vi "Init Plot Toolbar.vi"(8 "error in (no error)":errorcluster, 11 "Refs":T1) -> (0 "error out":errorcluster, 3 "Refs (dup)":T1)   [LabVIEW 2021, in "RocketPlot.lvlib"]
uses:
  RocketPlot.lvlib
  TypeDefs/Plot UI references.ctl
  Classes/RocketPlotHandle/RocketPlotHandle.lvclass
  <userlib>/bjustice/TipStripOOPanel/Classes/TipPanelHandle/TipPanelHandle.lvclass
  TypeDefs/Plot top row.ctl
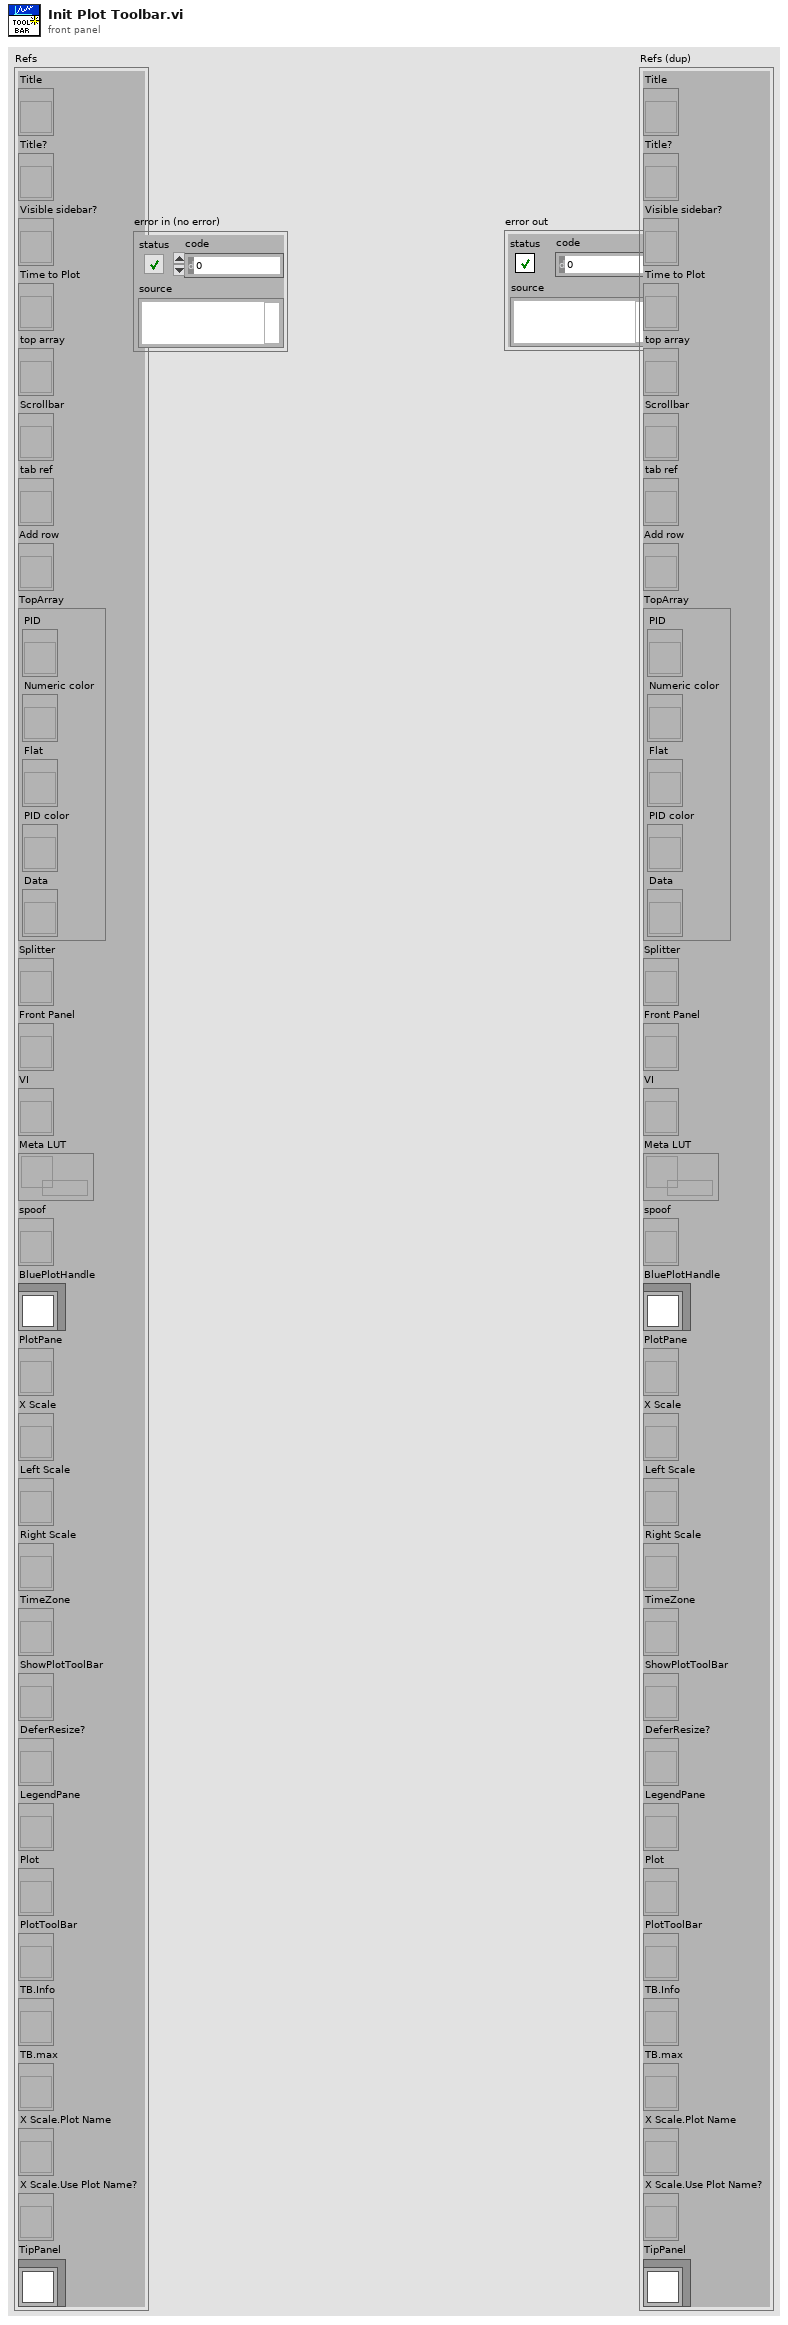
[diagram p1: front panel]
types:
  T1 = typedef "RocketPlot.lvlib/Plot UI references.ctl" = cluster{"Title":refnum<vi>, "Title?":refnum<vi>, "Visible sidebar?":refnum<vi>, "Time to Plot":refnum<vi>, "top array":refnum<vi>, "Scrollbar":refnum<vi>, "tab ref":refnum<vi>, "Add row":refnum<vi>, "TopArray":cluster{"PID":refnum<vi>, "Numeric color":refnum<vi>, "Flat":refnum<vi>, "PID color":refnum<vi>, "Data":refnum<vi>}, "Splitter":refnum<vi>, "Front Panel":refnum<vi>, "VI":refnum<vi>, "Meta LUT":refnum<data-value>, "spoof":refnum<vi>, "BluePlotHandle":refnum<class "RocketPlotHandle.lvclass">, "PlotPane":refnum<vi>, "X Scale":refnum<vi>, "Left Scale":refnum<vi>, "Right Scale":refnum<vi>, "TimeZone":refnum<vi>, "ShowPlotToolBar":refnum<vi>, "DeferResize?":refnum<vi>, "LegendPane":refnum<vi>, "Plot":refnum<vi>, "PlotToolBar":refnum<vi>, "TB.Info":refnum<vi>, "TB.max":refnum<vi>, "X Scale.Plot Name":refnum<vi>, "X Scale.Use Plot Name?":refnum<vi>, "TipPanel":refnum<class "TipPanelHandle.lvclass">}
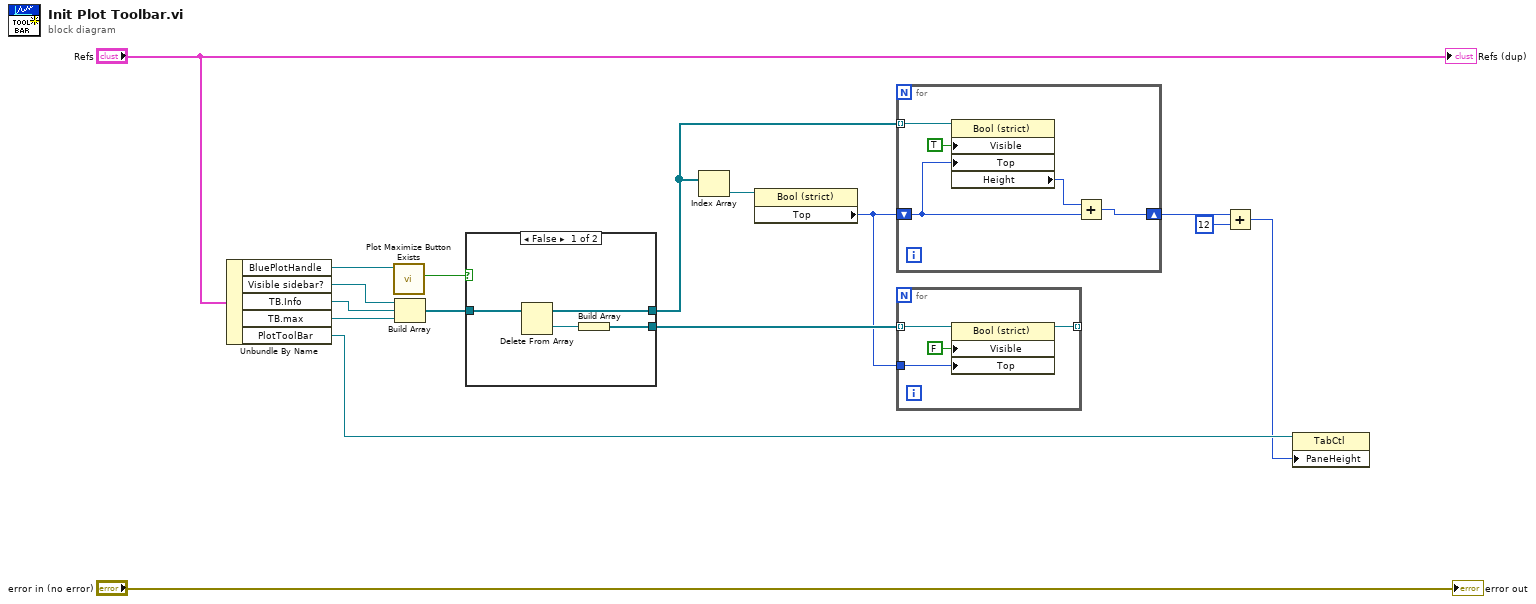
[diagram p0: block diagram]
diagram:
  n1 = Unbundle By Name("Refs") -> ("BluePlotHandle"=w12:refnum<class "RocketPlotHandle.lvclass">, "Visible sidebar?"=w15:refnum<vi>, "TB.Info"=w14:refnum<vi>, "TB.max"=w13:refnum<vi>, "PlotToolBar"=w4:refnum<vi>)
  n2 = call-dynamic "Plot Maximize Button Exists.vi"("BluePlotHandle in"=w12) -> ("Plot Maximize Button exists?"=w11:bool)  [unwired: 8 in, 2 out]
  n3 = Build Array(w15, w14, w13) -> (w10:refnum<vi>[])
  n4 = case shown="False" w11 {
    tunnel: w10 -> [w20 w21]
    tunnel: [w18 w21] -> w7
    tunnel: [w17 _] -> w9
    frame False {
      n5 = Delete From Array(array=w20) -> (deleted portion=w19:refnum<vi>, array with subset deleted=w18:refnum<vi>[])  [unwired: 2 in]
      n6 = Build Array(w19) -> (w17:refnum<vi>[])
    }
    frame True {
    }
  }
  n7 = Index Array(array=w7) -> (element=w8:refnum<vi>)  [unwired: 1 in]
  n8 = property class="Bool (strict)"(reference=w8) -> ("Top"=w6:i32)  [unwired: 1 in, 2 out]
  n9 = for {
    tunnel: w7 -> [w26] mode=indexing
    shift-right: [w22] -> w2
    shift-left: w6 -> [w23]
    n10 = property class="Bool (strict)"(reference=w26, "Visible"=TRUE, "Top"=w23) -> ("Height"=w24:u32)  [unwired: 1 in, 2 out]
    n11 = Add(x=w24, y=w23) -> (x+y=w22:u32)
  }
  n12 = for {
    tunnel: w9 -> [w30] mode=indexing
    tunnel: w6 -> [w28]
    tunnel: [w27] -> _ mode=indexing
    n13 = property class="Bool (strict)"(reference=w30, "Visible"=FALSE, "Top"=w28) -> (reference out=w27:refnum<vi>)  [unwired: 1 in, 1 out]
  }
  n14 = Add(x=w2, y=u32 12) -> (x+y=w1:u32)
  n15 = property class="TabCtl"(reference=w4, "PaneHeight"=w1) -> ()  [unwired: 1 in, 2 out]
  "error out" <- "error in (no error)"
  "Refs (dup)" <- "Refs"
